vi "CreateShutdownXML.vi"() -> (0 "XML":string)   [LabVIEW 2012]
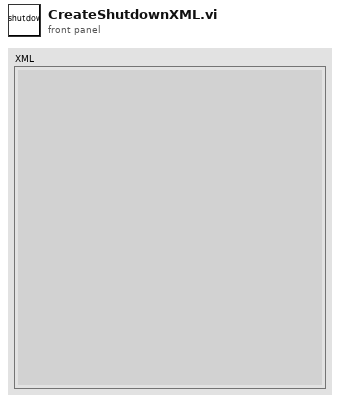
[diagram p1: front panel]
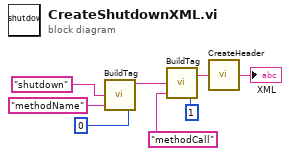
[diagram p0: block diagram]
diagram:
  n1 = call <userlib>:"BuildTag.vi"("Indent"=i8 0, "tag"="methodName", "value"="shutdown" ("MethodName")) -> ("string out"=w1:string)  [unwired: 1 in]
  n2 = call <userlib>:"BuildTag.vi"("Indent"=i8 1, "tag"="methodCall", "value"=w1) -> ("string out"=w3:string)  [unwired: 1 in]
  n3 = call <userlib>:"CreateHeader.vi"("Content"=w3) -> ("XML"=→"XML":string)
